vi "Normal Log List.vi"(8 "error in (no error)":errorcluster, 10 "log":string[](array[string]), 11 "Normal Log in":refnum<class "Normal Log.lvclass">) -> (0 "error out":errorcluster, 3 "Normal Log out":refnum<class "Normal Log.lvclass">)   [LabVIEW 2020, in "Normal Log.lvlib" / "Normal Log.lvclass"]
uses:
  Normal Log.lvclass
  Normal Log Messages/Append Log List Msg/Append Log List Msg.lvclass
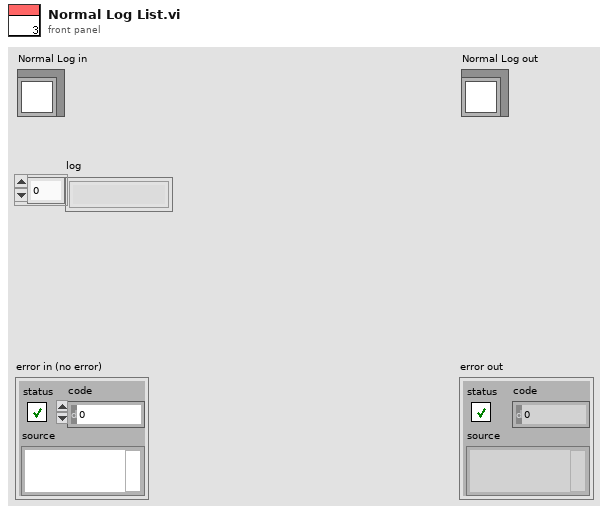
[diagram p1: front panel]
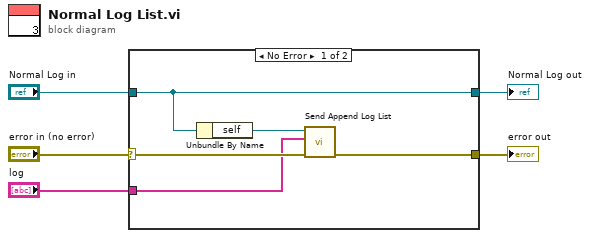
[diagram p0: block diagram]
diagram:
  n1 = case shown="No Error" "error in (no error)" {
    selector: "error in (no error)" -> [w9 w12]
    tunnel: "log" -> [w6 _]
    tunnel: "Normal Log in" -> [w10 w11]
    tunnel: [w8 w12] -> w2
    tunnel: [w10 w11] -> w1
    frame No Error {
      n2 = Unbundle By Name(w10) -> ("self"=w7:refnum<class "Message Enqueuer.lvclass">)
      n3 = call "Send Append Log List.vi"("error in (no error)"=w9, "log list"=w6, "Message Enqueuer"=w7) -> ("error out"=w8:errorcluster)  [unwired: 7 in, 1 out]
    }
    frame Error {
    }
  }
  "error out" <- w2
  "Normal Log out" <- w1
